vi "PlaceSnake.vi"(8 "error in (no error)":errorcluster, 9 "Tail col":i32, 10 "Tail row":i32, 11 "Board in":T1[][](array[typedef])) -> (0 "error out":errorcluster, 1 "Tail Position":cluster{"row":i32, "col":i32}, 2 "Head Position":cluster{"row":i32, "col":i32}, 3 "Board out":T1[][](array[typedef]))   [LabVIEW 2020]
doc: "Places a snake facing right. Tail at indicated position. Provides positions for head and tail. \nReturns (-1,-1) in case that snake cannot be placed."
uses:
  TypeDef/tiles-key.ctl
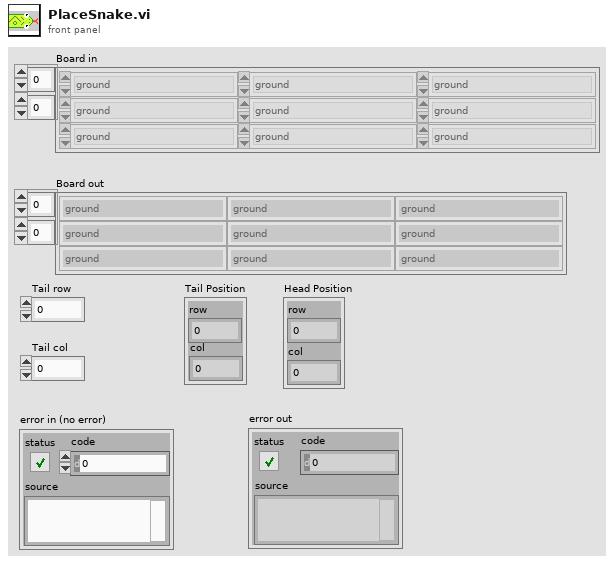
[diagram p1: front panel]
types:
  T1 = typedef "tiles-key.ctl" = enum16{"ground", "wall", "head (right)", "head (up)", "head (left)", "head (down)", "L-turn (right-up)", "L-turn (up-left)", "L-turn (left-down)", "L-turn (down-right)", "body (right)", "body (up)", "body (left)", "body (down)", "R-turn (right-down)", "R-turn (up-right)", "R-turn (left-up)", "R-turn (down-left)", "tail (right)", "tail (up)", "tail (left)", "tail (down)", "dead head (right)", "dead head (up)", "dead head (left)", "dead head (down)", "dead L-turn (right-up)", "dead L-turn (up-left)", "dead L-turn (left-down)", "dead L-turn (down-right)", "dead body (right)", "dead body (up)", "dead body (left)", "dead body (down)", "dead R-turn (right-down)", "dead R-turn (up-right)", "dead R-turn (left-up)", "dead R-turn (down-left)", "dead tail (right)", "dead tail (up)", "dead tail (left)", "dead tail (down)", "target red", "target blue", "target yellow", "target green"}
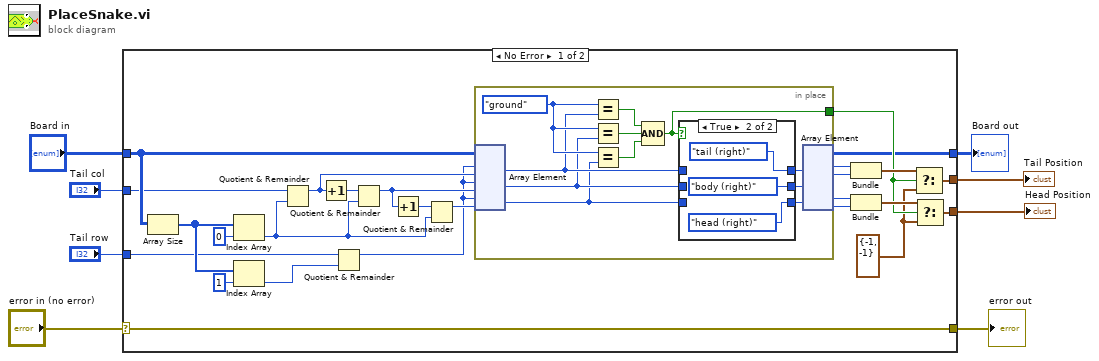
[diagram p0: block diagram]
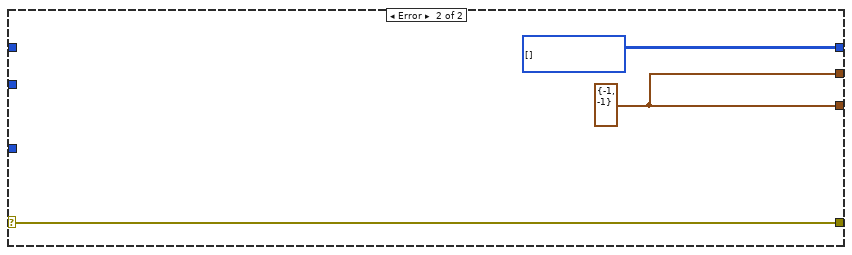
[diagram p3: hidden frame]
diagram:
  n1 = case shown="No Error" "error in (no error)" {
    selector: "error in (no error)" -> [w20 w54]
    tunnel: "Board in" -> [w23 _]
    tunnel: "Tail col" -> [w22 _]
    tunnel: "Tail row" -> [w21 _]
    tunnel: [w20 w54] -> w6
    tunnel: [w19 w53] -> w5
    tunnel: [w18 w52] -> w4
    tunnel: [w17 w52] -> w3
    frame No Error {
      w30 = cluster{i32, i32} {-1, -1} ("f")
      n2 = Array Size(array=w23) -> (size(s)=w27:i32[])
      n3 = Index Array(array=w27, index=0) -> (element=w25:i32)
      n4 = Index Array(array=w27, index=1) -> (element=w24:i32)
      n5 = Quotient & Remainder(x=w22, y=w25) -> (x-y*floor(x/y)=w10:i32)  [unwired: 1 out]
      n6 = Increment(x=w10) -> (x+1=w34:i32)
      n7 = Quotient & Remainder(x=w21, y=w24) -> (x-y*floor(x/y)=w9:i32)  [unwired: 1 out]
      n8 = Quotient & Remainder(x=w34, y=w25) -> (x-y*floor(x/y)=w11:i32)  [unwired: 1 out]
      n9 = Increment(x=w11) -> (x+1=w29:i32)
      n10 = Quotient & Remainder(x=w29, y=w25) -> (x-y*floor(x/y)=w12:i32)  [unwired: 1 out]
      n11 = in-place {
        in-place-border: [w35] -> w31
        w45 = tiles-key."ground" ("new element/subarray")
        n12 = in-place-array #1(w23, w9, w10, w9, w11, w9, w12) -> (w38:T1, w37:T1, w36:T1)
        n13 = Equal?(x=w45, y=w38) -> (x = y?=w44:bool)
        n14 = Equal?(x=w45, y=w37) -> (x = y?=w43:bool)
        n15 = Equal?(x=w45, y=w36) -> (x = y?=w42:bool)
        n16 = Compound Arithmetic op=AND(w44, w43, w42) -> (w35:bool)
        n17 = case shown="True" w35 {
          tunnel: [w48 tiles-key."tail (right)" ("new element/subarray")] -> w41
          tunnel: [w47 tiles-key."body (right)" ("new element/subarray")] -> w40
          tunnel: [w46 tiles-key."head (right)" ("new element/subarray")] -> w39
          tunnel: w38 -> [w48 _]
          tunnel: w37 -> [w47 _]
          tunnel: w36 -> [w46 _]
          frame False {
          }
          frame True {
          }
        }
        n18 = in-place-array #1(w41, w40, w39) -> (w19:T1[][], w16:i32, w15:i32, w14:i32, w13:i32)  [unwired: 2 out]
      }
      n19 = Bundle(w16, w15) -> (w33:cluster{i32, i32})  [unwired: 1 in]
      n20 = Bundle(w14, w13) -> (w32:cluster{i32, i32})  [unwired: 1 in]
      n21 = Select(t=w33, s=w31, f=w30) -> (s? t:f=w18:cluster{i32, i32})
      n22 = Select(t=w32, s=w31, f=w30) -> (s? t:f=w17:cluster{i32, i32})
    }
    frame Error {
      w52 = cluster{i32, i32} {-1, -1} ("f")
      w53 = T1[][] [] items=["ground", "wall", "head (right)", "head (up)", "head (left)", "head (down)", "L-turn (right-up)", "L-turn (up-left)", "L-turn (left-down)", "L-turn (down-right)", "body (right)", "body (up)", "body (left)", "body (down)", "R-turn (right-down)", "R-turn (up-right)", "R-turn (left-up)", "R-turn (down-left)", "tail (right)", "tail (up)", "tail (left)", "tail (down)", "dead head (right)", "dead head (up)", "dead head (left)", "dead head (down)", "dead L-turn (right-up)", "dead L-turn (up-left)", "dead L-turn (left-down)", "dead L-turn (down-right)", "dead body (right)", "dead body (up)", "dead body (left)", "dead body (down)", "dead R-turn (right-down)", "dead R-turn (up-right)", "dead R-turn (left-up)", "dead R-turn (down-left)", "dead tail (right)", "dead tail (up)", "dead tail (left)", "dead tail (down)", "target red", "target blue", "target yellow", "target green"] ("Board in")
    }
  }
  "error out" <- w6
  "Board out" <- w5
  "Tail Position" <- w4
  "Head Position" <- w3
